vi "String to Array of Characters.vi"(11 "String":string) -> (3 "Array of Characters":string[](array[string]))   [LabVIEW 2024, in "Wordle Engine.lvlib"]
doc: "Converts a string to an array of the single characters in that string. For example, the string \"dog\" would be converted to an array of three elements: \"d\", \"o\", and \"g\"."
uses:
  Libraries/Wordle Engine/Wordle Engine.lvlib
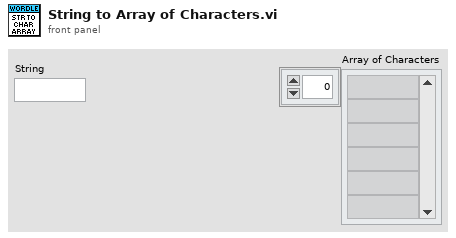
[diagram p1: front panel]
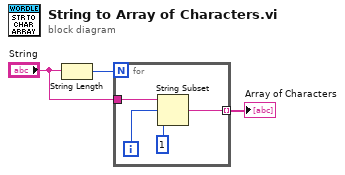
[diagram p0: block diagram]
diagram:
  n1 = String Length(string="String") -> (length=w3:i32)
  n2 = for {
    N: w3 -> [_]
    tunnel: "String" -> [w7]
    tunnel: [w4] -> w1 mode=indexing
    i -> [w6]
    n3 = String Subset(string=w7, offset (0)=w6, length (rest)=1 ("length (rest)")) -> (substring=w4:string)
  }
  "Array of Characters" <- w1
